vi "SUR.vi"(5 "Time (s)":dbl, 7 "Change Reactivity (dk)":dbl, 11 "input cluster":T1) -> (3 "SUR (DPM)":dbl)   [LabVIEW 2019]
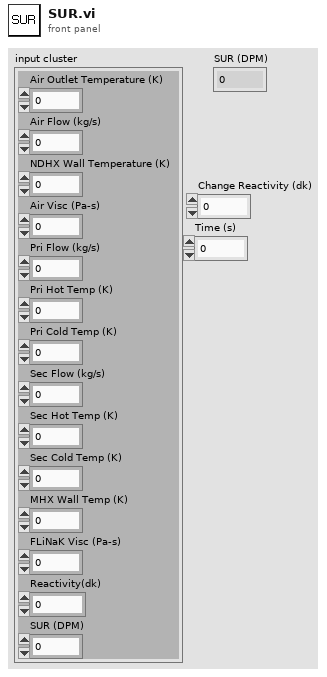
[diagram p1: front panel]
types:
  T1 = cluster{"Air Outlet Temperature (K)":dbl, "Air Flow (kg/s)":dbl, "NDHX Wall Temperature (K)":dbl, "Air Visc (Pa-s)":dbl, "Pri Flow (kg/s)":dbl, "Pri Hot Temp (K)":dbl, "Pri Cold Temp (K)":dbl, "Sec Flow (kg/s)":dbl, "Sec Hot Temp (K)":dbl, "Sec Cold Temp (K)":dbl, "MHX Wall Temp (K)":dbl, "FLiNaK Visc (Pa-s)":dbl, "Reactivity(dk)":dbl, "SUR (DPM)":dbl}
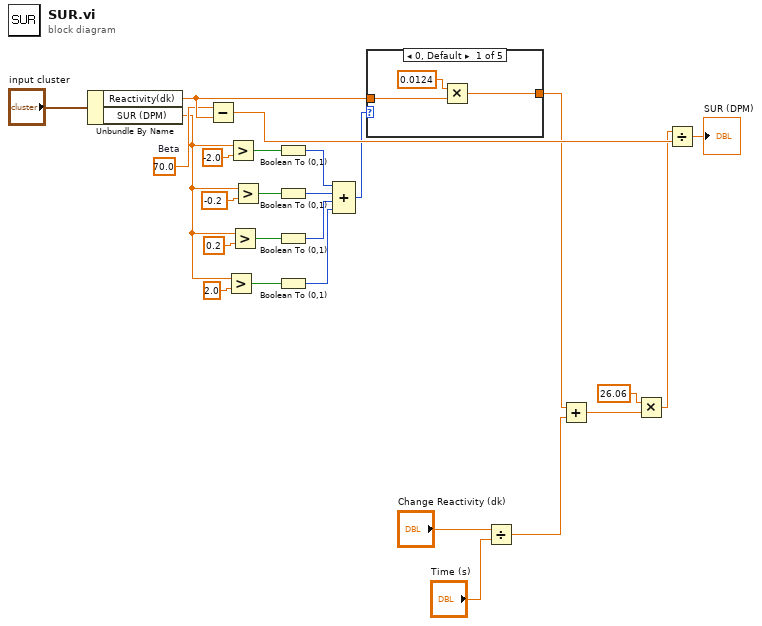
[diagram p0: block diagram]
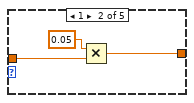
[diagram p2: hidden frame]
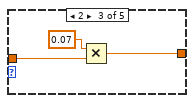
[diagram p3: hidden frame]
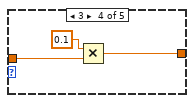
[diagram p4: hidden frame]
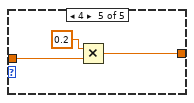
[diagram p5: hidden frame]
diagram:
  w23 = 70.0  # Beta
  n1 = Unbundle By Name("input cluster") -> ("Reactivity(dk)"=w25:dbl, "SUR (DPM)"=w14:dbl)
  n2 = Subtract(x=w23, y=w25) -> (x-y=w22:dbl)
  n3 = Greater?(x=w14, y=2.0) -> (0:w8:bool)
  n4 = Greater?(x=w14, y=-2.0) -> (0:w12:bool)
  n5 = Greater?(x=w14, y=0.2) -> (0:w9:bool)
  n6 = Greater?(x=w14, y=-0.2) -> (0:w10:bool)
  n7 = Boolean To (0,1)(Boolean=w12) -> (0, 1=w11:i16)
  n8 = Boolean To (0,1)(Boolean=w10) -> (0, 1=w7:i16)
  n9 = Boolean To (0,1)(Boolean=w9) -> (0, 1=w6:i16)
  n10 = Boolean To (0,1)(Boolean=w8) -> (0, 1=w5:i16)
  n11 = Compound Arithmetic op=ADD(w11, w7, w6, w5) -> (w4:i16)
  n12 = case shown="0, Default" w4 {
    tunnel: w25 -> [w28 w32 w35 w38 w41]
    tunnel: [w29 w30 w33 w36 w39] -> w20
    frame 0, Default {
      n13 = Multiply(x=0.0124, y=w28) -> (x*y=w29:dbl)
    }
    frame 1 {
      n14 = Multiply(x=0.05, y=w32) -> (x*y=w30:dbl)
    }
    frame 2 {
      n15 = Multiply(x=0.07, y=w35) -> (x*y=w33:dbl)
    }
    frame 3 {
      n16 = Multiply(x=0.1, y=w38) -> (x*y=w36:dbl)
    }
    frame 4 {
      n17 = Multiply(x=0.2, y=w41) -> (x*y=w39:dbl)
    }
  }
  n18 = Divide(x="Change Reactivity (dk)", y="Time (s)") -> (x/y=w1:dbl)
  n19 = Add(x=w20, y=w1) -> (x+y=w19:dbl)
  n20 = Multiply(x=26.06, y=w19) -> (x*y=w21:dbl)
  n21 = Divide(x=w21, y=w22) -> (x/y=→"SUR (DPM)":dbl)
